vi "ExecuteRunOperation.vi"(8 "error in (no error)":errorcluster, 9 "Inputs":string[](array[string]), 10 "CoreOperation.lvclass":refnum<class "CoreOperation.lvclass">, 11 "Logger in":refnum<class "Logger.lvclass">) -> (0 "error out":errorcluster, 2 "Output/Failure":string, 3 "CLI Process Return Code":i32)   [LabVIEW 2014]
uses:
  Logger/Logger.lvclass
  CoreOperation/CoreOperation.lvclass
  OperationErrorType.ctl
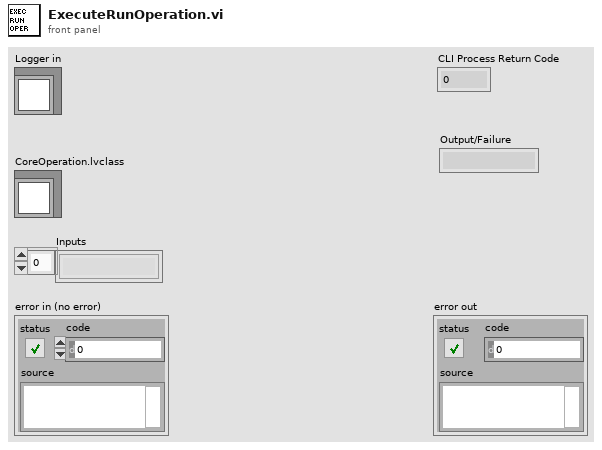
[diagram p1: front panel]
types:
  T1 = typedef "OperationErrorType.ctl" = enum16{"RequiredArgumentMissing", "UnknownArguments", "LoggerSetMultipleTimes", "OperationBrokenError"}
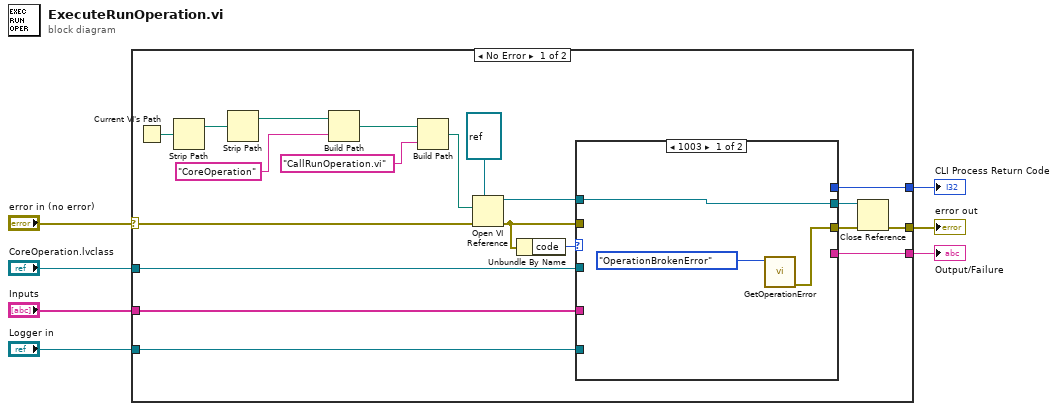
[diagram p0: block diagram]
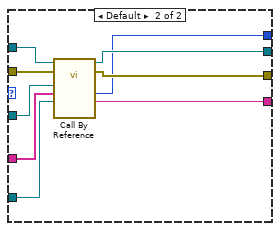
[diagram p2: hidden frame]
diagram:
  n1 = case shown="No Error" "error in (no error)" {
    selector: "error in (no error)" -> [w20 w40]
    tunnel: [w15 w40] -> w6
    tunnel: "CoreOperation.lvclass" -> [w14 _]
    tunnel: "Logger in" -> [w13 _]
    tunnel: "Inputs" -> [w12 _]
    tunnel: [w11 _] -> w2
    tunnel: [w10 _] -> w1
    frame No Error {
      n2 = Current VI's Path() -> (path=w27:path)
      n3 = Strip Path(path=w27) -> (stripped path=w26:path)  [unwired: 1 out]
      n4 = Strip Path(path=w26) -> (stripped path=w25:path)  [unwired: 1 out]
      n5 = Build Path(base path=w25, name or relative path="CoreOperation") -> (appended path=w23:path)
      n6 = Build Path(base path=w23, name or relative path="CallRunOperation.vi") -> (appended path=w21:path)
      n7 = Open VI Reference(type specifier VI Refnum (for type only)=refnum<vi> refnum, vi path=w21, error in (no error)=w20) -> (vi reference=w18:refnum<vi>, error out=w9:errorcluster)  [unwired: 3 in]
      n8 = Unbundle By Name(w9) -> ("code"=w8:i32)
      n9 = case shown="1003" w8 {
        tunnel: w18 -> [w30 w39]
        tunnel: w9 -> [_ w38]
        tunnel: [w30 w37] -> w17
        tunnel: [w29 w36] -> w16
        tunnel: w14 -> [_ w35]
        tunnel: w13 -> [_ w34]
        tunnel: w12 -> [_ w33]
        tunnel: [_ w32] -> w11
        tunnel: [_ w31] -> w10
        frame 1003 {
          n10 = call "GetOperationError.vi"("Operation Error Type"=OperationErrorType."OperationBrokenError") -> ("error out"=w29:errorcluster)  [unwired: 10 in]
        }
        frame Default {
          n11 = call-by-ref "?"(reference=w39, error in=w38, "Logger"=w34, "Inputs"=w33, "CoreOperation in"=w35) -> (reference out=w37:refnum<vi>, error out=w36:errorcluster, "Output/Failure"=w32:string, "CLI Process Return Code"=w31:i32)  [unwired: 4 in, 1 out]
        }
      }
      n12 = Close Reference(reference=w17, error in (no error)=w16) -> (error out=w15:errorcluster)
    }
    frame Error {
    }
  }
  "Output/Failure" <- w2
  "CLI Process Return Code" <- w1
  "error out" <- w6
